vi "Get Node Children Data.vi"(8 "error in (no error)":errorcluster, 10 "Node Path (parent, child)":string[](array[string]), 11 "Tree Map Handle In":T4) -> (0 "error out":errorcluster, 1 "Node Exists?":bool, 2 "tree node data map":T1, 3 "Tree Map Handle out":T4)   [LabVIEW 2020, in "Blue Tree Map OpenSource.lvlib"]
doc: "This will return the node data for all children of the specified node path.\nNote that the children tree path names represent the returned map keys."
uses:
  Blue Tree Map OpenSource.lvlib
  Typedefs/Tree Map Handle.ctl
  Typedefs/Tree Map.ctl
  Typedefs/Tree Map Data.ctl
  Typedefs/Tree Node Data.ctl
  Typedefs/Attribute Map.ctl
  Typedefs/Tree Node Data Map.ctl
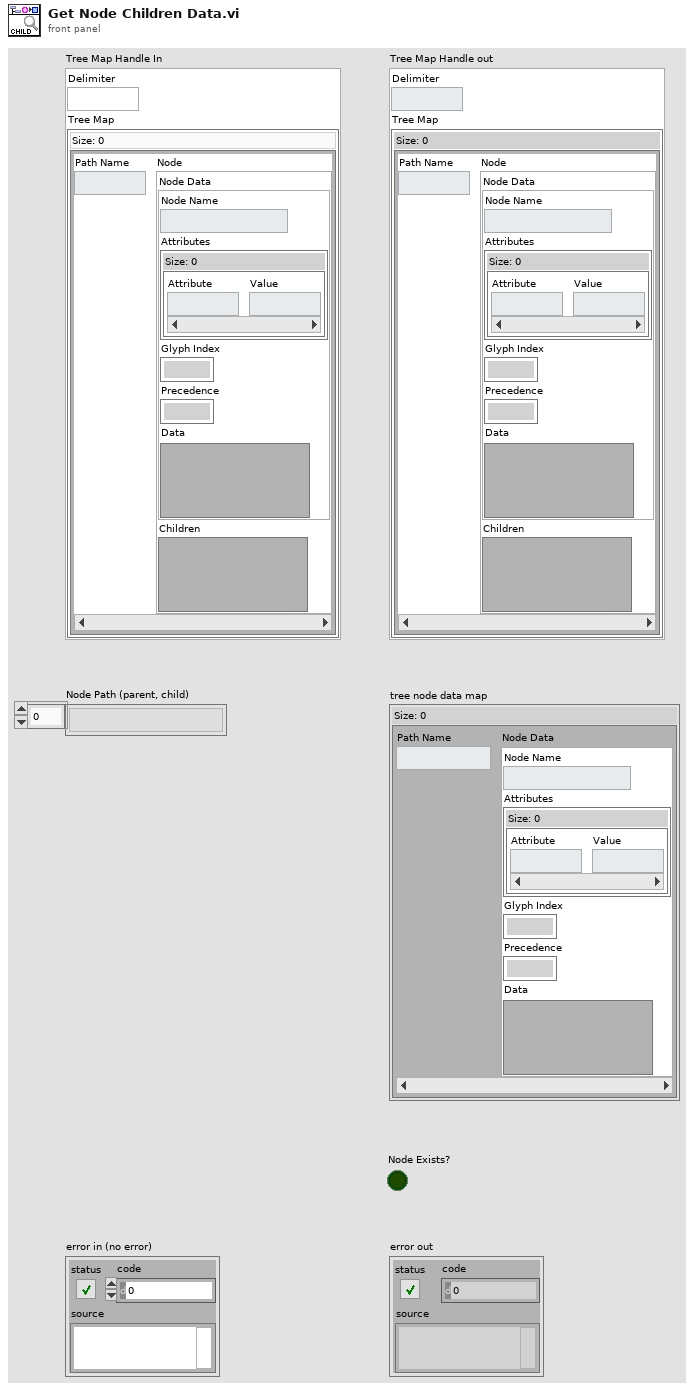
[diagram p1: front panel]
types:
  T1 = typedef "Blue Tree Map OpenSource.lvlib/Tree Node Data Map.ctl" = map{string, T2}
  T2 = typedef "Blue Tree Map OpenSource.lvlib/Tree Node Data.ctl" = cluster{"Node Name":string, "Attributes":T3, "Glyph Index":i32, "Precedence":i32, "Data":variant}
  T3 = typedef "Blue Tree Map OpenSource.lvlib/Attribute Map.ctl" = map{string, string}
  T4 = typedef "Blue Tree Map OpenSource.lvlib/Tree Map Handle.ctl" = cluster{"Delimiter":string, "Tree Map":T5}
  T5 = typedef "Blue Tree Map OpenSource.lvlib/Tree Map.ctl" = map{string, T6}
  T6 = typedef "Blue Tree Map OpenSource.lvlib/Tree Map Data.ctl" = cluster{"Node Data":T2, "Children":variant}
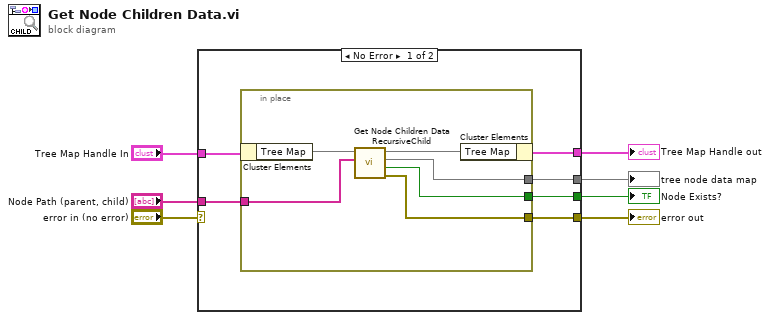
[diagram p0: block diagram]
diagram:
  n1 = case shown="No Error" "error in (no error)" {
    selector: "error in (no error)" -> [_ w21]
    tunnel: "Tree Map Handle In" -> [w13 w20]
    tunnel: "Node Path (parent, child)" -> [w12 _]
    tunnel: [w11 _] -> w5
    tunnel: [w10 w20] -> w4
    tunnel: [w9 w21] -> w3
    tunnel: [w8 _] -> w1
    frame No Error {
      n2 = in-place {
        in-place-border: w12 -> [w17]
        in-place-border: [w15] -> w8
        in-place-border: [w16] -> w11
        in-place-border: [w14] -> w9
        n3 = in-place-cluster #1(w13) -> ("Tree Map"=w19:T5)
        n4 = call "Get Node Children Data RecursiveChild.vi"("Node Path (parent, child)"=w17, "Tree Map In"=w19) -> ("error out"=w14:errorcluster, "Node Exists?"=w16:bool, "tree node data map"=w15:T1, "Tree Map Out"=w18:T5)  [unwired: 6 in]
        n5 = in-place-cluster #1("Tree Map"=w18) -> (w10:T4)
      }
    }
    frame Error {
    }
  }
  "error out" <- w3
  "Tree Map Handle out" <- w4
  "Node Exists?" <- w5
  "tree node data map" <- w1
